vi "test.vi"() -> ()   [LabVIEW 2011]
uses:
  <vilib>/robotics/Steering/Wheel/NI_Robotics_Wheel.lvclass
  <vilib>/robotics/Steering/Mecanum Wheel/Create Mecanum Wheel.vi
  <vilib>/robotics/Steering/Mecanum Wheel/NI_Robotics_Mecanum Wheel.lvclass
  <vilib>/robotics/Steering/Steering Frame/NI_Robotics_Steering Frame.lvclass
  <vilib>/robotics/Steering/Mecanum Steering Frame/Create Mecanum Steering Frame.vi
  <vilib>/robotics/Steering/Mecanum Steering Frame/NI_Robotics_Mecanum Steering Frame.lvclass
  <vilib>/robotics/Utilities/Visualization/Steering Visualization/Steering Picture/Draw Steering Frame Options.ctl
  <vilib>/robotics/Utilities/Visualization/Steering Visualization/Steering Picture/NI_Robotics_Steering Picture.lvlib
  <vilib>/robotics/Steering/Steering Frame/Apply Steering Frame Velocity to Wheels.vi
  <vilib>/robotics/Steering/Wheel/Wheel Parameters.ctl
  <vilib>/robotics/Steering/Wheel/Rotation Direction.ctl
  <vilib>/Utility/inputDevices.llb/mouseAcquire.vi
  <vilib>/Utility/inputDevices.llb/closeMouse.vi
panel:
  in  "key mode":enum16{"RELATIVE", "ABSOLUTE"}(ring)=enum."ABSOLUTE"
  out "button info":T1
  out "error out":errorcluster
  in  "stop":bool
  out "picture":picture
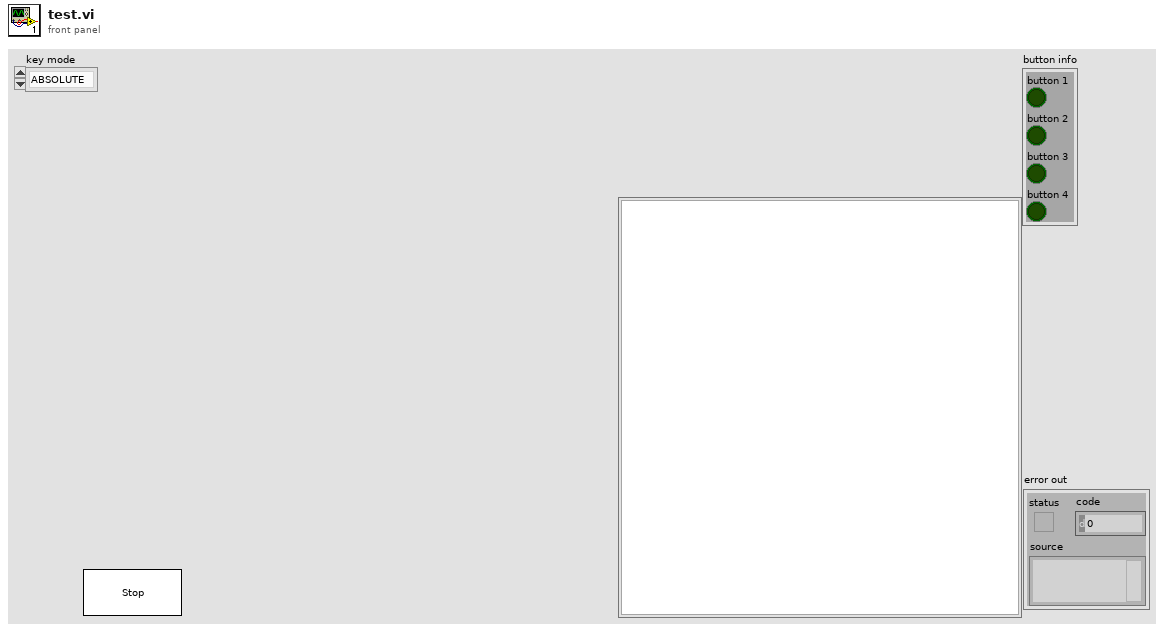
[diagram p1: front panel]
types:
  T1 = cluster{"button 1":bool, "button 2":bool, "button 3":bool, "button 4":bool}
  T2 = typedef "NI_Robotics_Steering Picture.lvlib/Draw Steering Frame Options.ctl" = cluster{"draw wheel states?":bool, "highlight wheel index":i32, "pixels per unit":dbl, "draw forward velocity?":bool, "velocity scale":dbl}
  T3 = typedef "NI_Robotics_Wheel.lvclass/Wheel Parameters.ctl" = cluster{"wheel radius":dbl, "gear ratio":dbl, "forward rotation direction":T4}
  T4 = typedef "NI_Robotics_Wheel.lvclass/Rotation Direction.ctl" = enum16{"Clockwise", "Counterclockwise"}
  T5 = cluster{"Horizontal":i32, "Vertical":i32, "Scrolling":i32}
  T6 = cluster{"mecanum wheel out":refnum<class "NI_Robotics_Mecanum Wheel.lvclass">, "mecanum wheel out":refnum<class "NI_Robotics_Mecanum Wheel.lvclass">, "mecanum wheel out":refnum<class "NI_Robotics_Mecanum Wheel.lvclass">, "mecanum wheel out":refnum<class "NI_Robotics_Mecanum Wheel.lvclass">}
  T7 = typedef "LVBoundsTypeDef.ctl" = cluster{"Width":u32, "Height":u32}
  T8 = typedef "NI_Robotics_Wheel.lvclass/Wheel State.ctl" = cluster{"wheel name":string, "forward angular velocity":dbl, "caster angular velocity":dbl, "caster wheel angle (rad)":dbl, "steering angle (rad)":dbl}
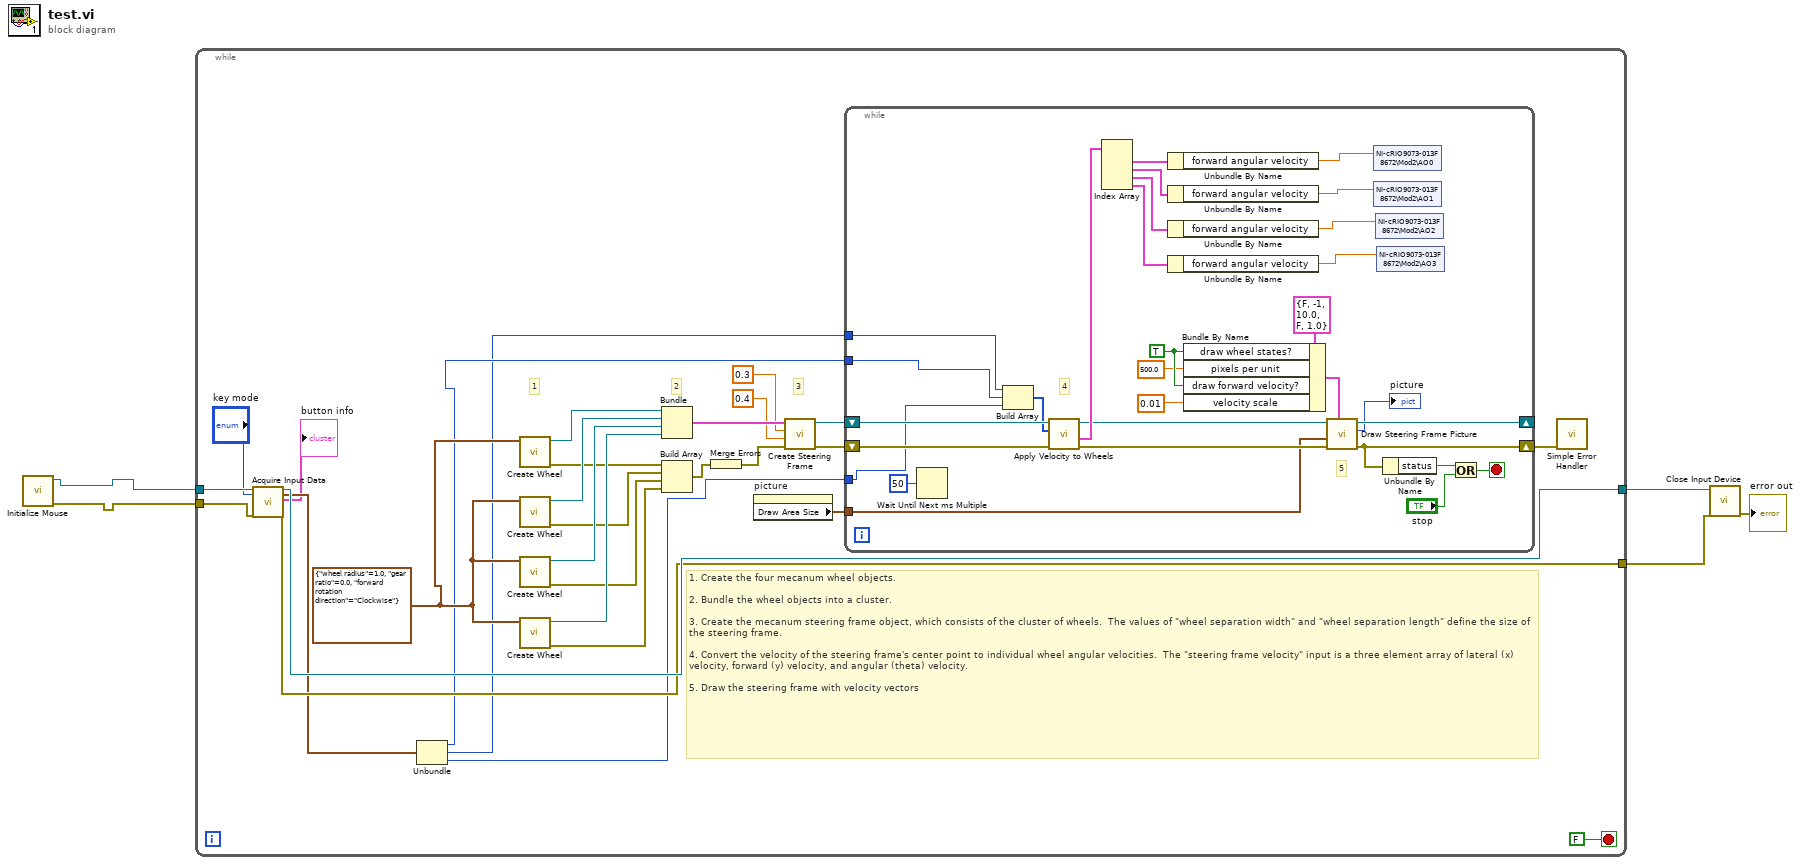
[diagram p0: block diagram]
diagram:
  n1 = call <vilib>:"Initialize Mouse.vi"() -> ("error out"=w1:errorcluster, "device ID"=w2:refnum<k1>)  [unwired: 10 in]
  n2 = while {
    tunnel: w2 -> [w17]
    tunnel: w1 -> [w16]
    tunnel: [w15] -> w5
    tunnel: [w14] -> w4
    stop <- FALSE stop-if-true
    w11 = T3 {"wheel radius"=1.0, "gear ratio"=0.0, "forward rotation direction"=enum."Clockwise"} ("wheel parameters")
    # "3"
    # "2"
    # "1"
    # "1. Create the four mecanum wheel objects.\n\n2. Bundle the wheel objects into a cluster.\n\n3. Create the mecanum steering frame object, which consists of the cluster of wheels.  The values of \"wheel separation width\" and \"wheel separation length\" define the size of the steering frame.\n\n4. Convert the velocity of the steering frame's center point to individual wheel angular velocities.  The \"steering frame velocity\" input is a three element array of lateral (x) velocity, forward (y) velocity, and angular (theta) velocity.\n\n5. Draw the steering frame with velocity vectors"
    n3 = call-poly <vilib>:"Acquire Input Data.vi"("device ID"=w17, "key mode"="key mode", "error in (no error)"=w16) -> ("device ID"=w15:refnum<k1>, "axis info"=w12:T5, "button info"=→"button info":T1, "error out"=w14:errorcluster)  [unwired: 13 in]
    n4 = Unbundle(w12) -> ("Horizontal"=w9:i32, "Vertical"=w8:i32, "Scrolling"=w7:i32)
    n5 = call-poly <vilib>:"Create Wheel.vi"("wheel parameters"=w11) -> ("error out"=w24:errorcluster, "mecanum wheel out"=w34:refnum<class "NI_Robotics_Mecanum Wheel.lvclass">)  [unwired: 9 in]
    n6 = call-poly <vilib>:"Create Wheel.vi"("wheel parameters"=w11) -> ("error out"=w23:errorcluster, "mecanum wheel out"=w33:refnum<class "NI_Robotics_Mecanum Wheel.lvclass">)  [unwired: 9 in]
    n7 = call-poly <vilib>:"Create Wheel.vi"("wheel parameters"=w11) -> ("error out"=w22:errorcluster, "mecanum wheel out"=w32:refnum<class "NI_Robotics_Mecanum Wheel.lvclass">)  [unwired: 9 in]
    n8 = call-poly <vilib>:"Create Wheel.vi"("wheel parameters"=w11) -> ("error out"=w20:errorcluster, "mecanum wheel out"=w31:refnum<class "NI_Robotics_Mecanum Wheel.lvclass">)  [unwired: 9 in]
    n9 = Bundle("mecanum wheel out"=w34, "mecanum wheel out"=w33, "mecanum wheel out"=w32, "mecanum wheel out"=w31) -> (w30:T6)  [unwired: 1 in]
    n10 = Build Array(w24, w23, w22, w20) -> (w21:errorcluster[])
    n11 = Merge Errors(w21) -> (w19:errorcluster)
    n12 = property on="picture" class="Pict"() -> ("Draw Area Size"=w18:T7)  [unwired: 2 in, 2 out]
    n13 = call-poly <vilib>:"Create Steering Frame.vi"("error in (no error)"=w19, "wheel separation length"=0.4, "wheel separation width"=0.3, "wheels"=w30) -> ("error out"=w26:errorcluster, "mecanum steering frame out"=w27:refnum<class "NI_Robotics_Mecanum Steering Frame.lvclass">)  [unwired: 6 in]
    n14 = while {
      shift-right: [w53] -> _
      shift-left: w27 -> [w55]
      shift-right: [w52] -> w25
      shift-left: w26 -> [w54]
      tunnel: w18 -> [w48]
      tunnel: w8 -> [w42]
      tunnel: w9 -> [w41]
      tunnel: w7 -> [w40]
      stop <- w57 stop-if-true
      w45 = TRUE ("draw wheel states")
      # "5"
      # "4"
      n15 = Wait Until Next ms Multiple(millisecond multiple=u32 50) -> ()  [unwired: 1 out]
      n16 = Build Array(w42, w41, w40) -> (w39:i32[])
      n17 = call-poly <vilib>:"Apply Velocity to Wheels.vi"("error in (no error)"=w54, "steering frame velocity"=w39, "steering frame in"=w55) -> ("error out"=w49:errorcluster, "calculated wheel states"=w56:T8[], "steering frame out"=w50:refnum<class "NI_Robotics_Mecanum Steering Frame.lvclass">)  [unwired: 5 in, 1 out]
      n18 = Index Array(array=w56) -> (element #1=w63:T8, element #2=w60:T8, element #3=w61:T8, element #4=w62:T8)  [unwired: 4 in]
      n19 = Unbundle By Name(w63) -> ("forward angular velocity"=w38:dbl)
      n20 = Unbundle By Name(w60) -> ("forward angular velocity"=w37:dbl)
      n21 = Unbundle By Name(w61) -> ("forward angular velocity"=w36:dbl)
      n22 = Unbundle By Name(w62) -> ("forward angular velocity"=w35:dbl)
      n23 = Bundle By Name(cluster=T2 {"draw wheel states?"=FALSE, "highlight wheel index"=-1, "pixels per unit"=10.0, "draw forward velocity?"=FALSE, "velocity scale"=1.0} ("draw options"), "draw wheel states?"=w45, "pixels per unit"=500.0 ("pixels per unit (10)"), "draw forward velocity?"=w45, "velocity scale"=0.01 ("velocity scale (1)")) -> (w43:T2)
      n24 = call <vilib>:"Draw Steering Frame Picture.vi"("drawing options"=w43, "error in (no error)"=w49, "picture draw area size (pixels)"=w48, "steering frame in"=w50) -> ("error out"=w52:errorcluster, "picture out"=→"picture":picture, "steering frame out"=w53:refnum<class "NI_Robotics_Mecanum Steering Frame.lvclass">)  [unwired: 5 in]
      n25 = shared-variable "NI-cRIO9073-013F8672\\Mod2\\AO0"(w38) -> ()  [unwired: 1 in, 1 out]
      n26 = shared-variable "NI-cRIO9073-013F8672\\Mod2\\AO1"(w37) -> ()  [unwired: 1 in, 1 out]
      n27 = shared-variable "NI-cRIO9073-013F8672\\Mod2\\AO2"(w36) -> ()  [unwired: 1 in, 1 out]
      n28 = shared-variable "NI-cRIO9073-013F8672\\Mod2\\AO3"(w35) -> ()  [unwired: 1 in, 1 out]
      n29 = Unbundle By Name(w52) -> ("status"=w59:bool)
      n30 = Or(x=w59, y="stop") -> (x .or. y?=w57:bool)
    }
    n31 = call <vilib>:"Simple Error Handler.vi"("error in (no error)"=w25) -> ()  [unwired: 4 in, 5 out]
  }
  n32 = call-poly <vilib>:"Close Input Device.vi"("error in (no error)"=w4, "device ID"=w5) -> ("error out"=→"error out":errorcluster)  [unwired: 8 in]
